vi "SubLaunch.vi"(8 "error in (no error)":errorcluster, 9 "ID":string, 10 "DeviceObj":refnum<class "Configurable Device.lvclass">, 11 "Controller in":refnum<class "Controller.lvclass">) -> (0 "error out":errorcluster, 3 "Controller out":refnum<class "Controller.lvclass">)   [LabVIEW 2018, in "Controller.lvlib" / "Controller.lvclass"]
doc: "Launches the devices. Devices are launched in parallel. All references to the devices are stored in the Enqueuer MAP and the data map which are both stored in DVRs. This is how we are able to do this in parallel."
uses:
  Controller.lvclass
  C:/Users/Labview/Documents/exscalabar_server/SuperActor/SuperActor.lvclass
  Devices/Configurable Device/Configurable Device.lvclass
  SuperActor/SuperActor.lvclass/SuperActor.ctl
  Messages/Update Device Configuration MSG/Update Device Configuration MSG.lvclass
  C:/Users/Labview/Documents/exscalabar_server/Controller/Messages/Device Configuration/Get Serialized Device Configuration MSG.lvclass
  reusable/Session APIs/File Access/Config Data/Config Data.lvclass
  Messages/Device Init CVT/Device Init CVT MSG.lvclass
  C:/Users/Labview/Documents/exscalabar_server/reusable/DAQ Device/Messages/Generic CVT Init/Generic Init CVT Message.lvclass
  Update Controller Data MSG.lvclass
  C:/Users/Labview/Documents/exscalabar_server/reusable/DAQ Device/Device/Generic Data Update Data MSG/Generic Update Data Message.lvclass
  Devices/Configurable Device/Configurable Device.lvclass/Configurable Device.ctl
  reusable/DAQ Device/Device/Device.lvclass
  C:/Program Files (x86)/National Instruments/LabVIEW 2018/vi.lib/ActorFramework/Actor/Actor.lvclass
  reusable/DAQ Device/Device/Generic Data Update Data MSG/Generic Update Data Message.lvclass/Generic Update Data Message.ctl
  reusable/DAQ Device/Device/Device.lvclass/Device.ctl
  SuperActor/Write ID.vi
  reusable/DAQ Device/Device/Generic Data Update Data MSG/Write ID.vi
  Devices/Configurable Device/Write ID.vi
  SuperActor/Read Config Session.vi
  reusable/Session APIs/File Access/Config Data/Read Array/Read String Array.vi
  <userlib>/_Session Fwk/Session - Root.lvclass
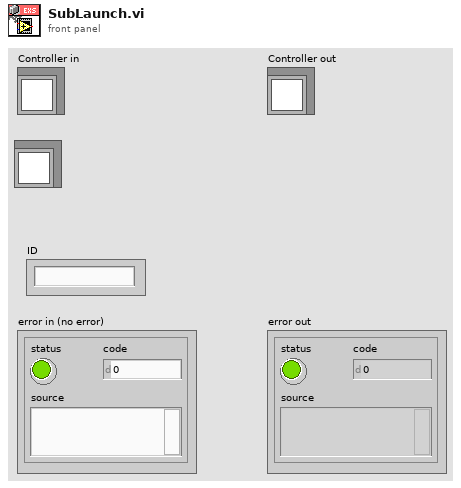
[diagram p1: front panel]
types:
  T1 = typedef "Session - Root.lvclass/Session Handle.ctl" = refnum<data-value>
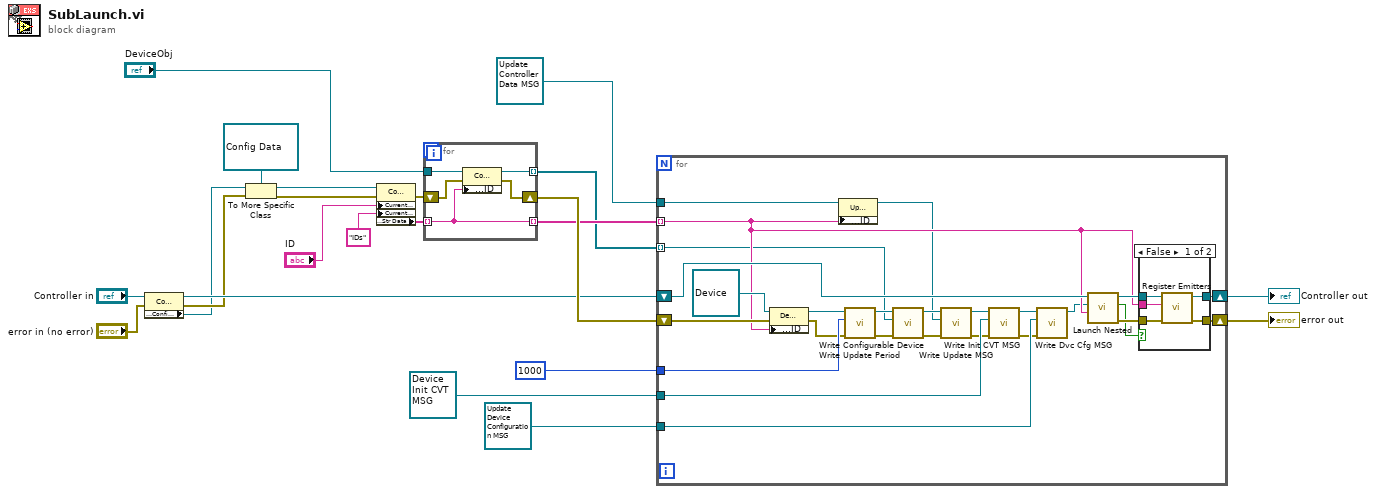
[diagram p0: block diagram]
diagram:
  n1 = property class="Controller"(reference="Controller in", error in="error in (no error)") -> (reference out=w15:refnum<class "Controller.lvclass">, error out=w13:errorcluster, "Accessors:Config Session"=w10:T1)
  n2 = To More Specific Class(target class=refnum<data-value> refnum, reference=w10, error in=w13) -> (specific class reference=w16:refnum<data-value>, error out=w19:errorcluster)
  n3 = property class="Config Data"(reference=w16, error in=w19, "Current Section"="ID", "Current Key"="IDs") -> (error out=w1:errorcluster, "Read Array Data:Str Data"=w2:string[])  [unwired: 1 out]
  n4 = for {
    tunnel: w2 -> [w25] mode=indexing
    tunnel: "DeviceObj" -> [w27]
    tunnel: [w26] -> w17 mode=indexing
    tunnel: [w25] -> w18 mode=indexing
    shift-right: [w24] -> w20
    shift-left: w1 -> [w23]
    n5 = property class="Configurable Device"(reference=w27, error in=w23, "Accessors:ID"=w25) -> (reference out=w26:refnum<class "Configurable Device.lvclass">, error out=w24:errorcluster)
  }
  n6 = for {
    tunnel: w17 -> [w36] mode=indexing
    shift-right: [w47] -> w6
    shift-left: w15 -> [w50]
    tunnel: refnum<class "Update Controller Data MSG.lvclass"> refnum ("Controller.lvlib:Update Data MSG") -> [w51]
    tunnel: w18 -> [w45] mode=indexing
    shift-right: [w46] -> w7
    shift-left: w20 -> [w52]
    tunnel: refnum<class "Device Init CVT MSG.lvclass"> refnum ("Controller.lvlib:Device Init CVT MSG") -> [w38]
    tunnel: refnum<class "Update Device Configuration MSG.lvclass"> refnum ("Controller:Update Device Configuration") -> [w39]
    tunnel: 1000 ("Update Period") -> [w35]
    n7 = property class="Device"(reference=refnum<class "Device.lvclass"> refnum ("DAQ Device.lvlib:Device"), error in=w52, "Accessors:ID"=w45) -> (reference out=w34:refnum<class "Device.lvclass">, error out=w33:errorcluster)
    n8 = property class="Update Data MSG"(reference=w51, "Accessors:ID"=w45) -> (reference out=w37:refnum<class "Update Controller Data MSG.lvclass">)  [unwired: 1 in, 1 out]
    n9 = call "Write Update Period.vi"("error in (no error)"=w33, "Update Period"=w35, "Device in"=w34) -> ("error out"=w32:errorcluster, "Device out"=w43:refnum<class "Device.lvclass">)  [unwired: 7 in]
    n10 = call "Write Configurable Device.vi"("error in (no error)"=w32, "Configurable Device"=w36, "Device in"=w43) -> ("error out"=w31:errorcluster, "Device out"=w42:refnum<class "Device.lvclass">)  [unwired: 7 in]
    n11 = call "Write Update MSG.vi"("error in (no error)"=w31, "DAQ Device.lvlib:Update Data MSG"=w37, "Device in"=w42) -> ("error out"=w30:errorcluster, "Device out"=w41:refnum<class "Device.lvclass">)  [unwired: 7 in]
    n12 = call "Write Init CVT MSG.vi"("error in (no error)"=w30, "DAQ Device.lvlib:Generic Init CVT Message"=w38, "Device in"=w41) -> ("error out"=w29:errorcluster, "Device out"=w40:refnum<class "Device.lvclass">)  [unwired: 7 in]
    n13 = call "Write Dvc Cfg MSG.vi"("error in (no error)"=w29, "DAQ Device.lvlib:Get Serialized Device Configuration MSG.lvclass"=w39, "Device in"=w40) -> ("Device out"=w28:refnum<class "Device.lvclass">)  [unwired: 7 in, 1 out]
    n14 = call "Launch Nested.vi"("ID"=w45, "Nested Actor"=w28, "Controller in"=w50) -> ("Error Out"=w48:errorcluster, "Launch Failure?"=w44:bool, "Controller out"=w49:refnum<class "Controller.lvclass">)  [unwired: 5 in, 1 out]
    n15 = case shown="False" w44 {
      tunnel: w49 -> [w58 w60]
      tunnel: w48 -> [w57 w59]
      tunnel: [w56 w60] -> w47
      tunnel: [w55 w59] -> w46
      tunnel: w45 -> [w54 _]
      frame False {
        n16 = call "Register Emitters.vi"("error in"=w57, "Emitter"=w54, "Controller in"=w58) -> ("error out"=w55:errorcluster, "Controller out"=w56:refnum<class "Controller.lvclass">)  [unwired: 7 in]
      }
      frame True {
      }
    }
  }
  "error out" <- w7
  "Controller out" <- w6
